vi "Choreo_DifferentialSample_Equals.vi"(9 "OtherChoreoSwerveSample":T1={"timestamp"=-999.0, "x"=0.0, "y"=0.0, "heading"=0.0, "velocityL"=0.0, "velocityR"=0.0, "angularVelocity"=0.0, "accelL"=0.0, "accelR"=0.0, "accelAngular"=0.0, "forceL"=0.0, "forceR"=0.0}, 11 "ChoreoSwerveSample":T1={"timestamp"=-999.0, "x"=0.0, "y"=0.0, "heading"=0.0, "velocityL"=0.0, "velocityR"=0.0, "angularVelocity"=0.0, "accelL"=0.0, "accelR"=0.0, "accelAngular"=0.0, "forceL"=0.0, "forceR"=0.0}) -> (3 "Equal":bool)   [LabVIEW 2019, in "ChoreoLib.lvlib"]
doc: "Determine if two Differential Trajectory Samples are equal\n\nInputs:\n -- ChoreoDifferentialSample - cluster - Differential sample.\n -- OtherChoreoDifferentialSample - cluster - Differential sample to compare.\n\nOutputs\"\n -- Equal - boolean - TRUE when the samples are the same"
uses:
  ChoreoLib.lvlib
  TypeDef/ChoreoDifferentialSample.ctl
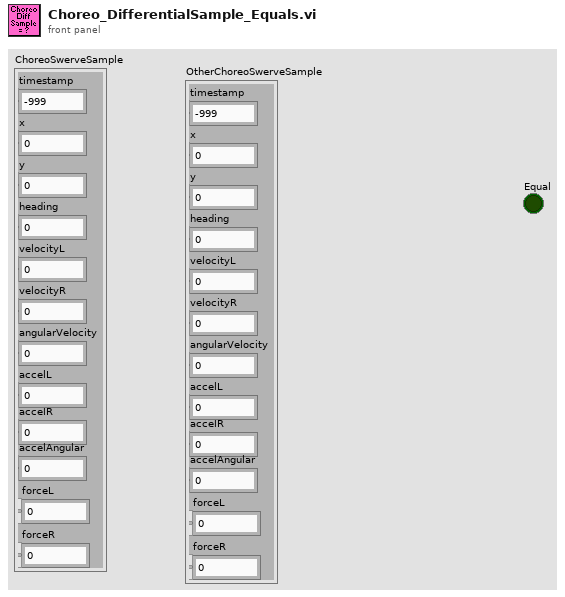
[diagram p1: front panel]
types:
  T1 = typedef "ChoreoLib.lvlib/ChoreoDifferentialSample.ctl" = cluster{"timestamp":dbl, "x":dbl, "y":dbl, "heading":dbl, "velocityL":dbl, "velocityR":dbl, "angularVelocity":dbl, "accelL":dbl, "accelR":dbl, "accelAngular":dbl, "forceL":dbl, "forceR":dbl}
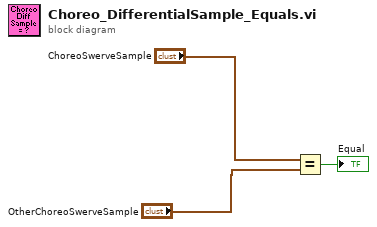
[diagram p0: block diagram]
diagram:
  n1 = Equal?(x="ChoreoSwerveSample", y="OtherChoreoSwerveSample") -> (x = y?=→"Equal":bool)
